vi "kalmanSeparatingObjects.vi"(1 "Detection Frame In":T1 {"robots_blue"."height" format="%+4.3f"; "robots_blue"."pixel_y" format="%+4.3f"; "robots_blue"."pixel_x" format="%+4.3f"; "robots_blue"."orientation" format="%+4.3f"; "robots_blue"."y" format="%+4.3f"; "robots_blue"."confidence" format="%4.3f"; "robots_blue"."x" format="%+4.3f"; "robots_yellow"."height" format="%+4.3f"; "robots_yellow"."pixel_y" format="%+4.3f"; "robots_yellow"."pixel_x" format="%+4.3f"; "robots_yellow"."orientation" format="%+4.3f"; "robots_yellow"."y" format="%+4.3f"; "robots_yellow"."confidence" format="%4.3f"; "robots_yellow"."x" format="%+4.3f"}, 3 "Time":enum16{"Azul", "Amarelo"}(ring) caption="Enum", 4 "Enable":bool) -> (15 "Detection Frame Out":T1 {"robots_blue"."height" format="%+4.3f"; "robots_blue"."pixel_y" format="%+4.3f"; "robots_blue"."pixel_x" format="%+4.3f"; "robots_blue"."orientation" format="%+4.3f"; "robots_blue"."y" format="%+4.3f"; "robots_blue"."confidence" format="%4.3f"; "robots_blue"."x" format="%+4.3f"; "robots_yellow"."height" format="%+4.3f"; "robots_yellow"."pixel_y" format="%+4.3f"; "robots_yellow"."pixel_x" format="%+4.3f"; "robots_yellow"."orientation" format="%+4.3f"; "robots_yellow"."y" format="%+4.3f"; "robots_yellow"."confidence" format="%4.3f"; "robots_yellow"."x" format="%+4.3f"})   [LabVIEW 2023, in "Vision.lvclass"]
uses:
  Vision.lvclass
  Old vision/Controls/SSL Detection Frame.ctl
  Old vision/Controls/SSL Detection Robot.ctl
  <vilib>/Analysis/Matrix/Datatypes/RealMatrix.ctl
  Old vision/Controls/SSL Detection Ball.ctl
  <vilib>/Analysis/Matrix/NI_Matrix.lvlib
panel:
  out "error out":errorcluster
  in  "error in (no error)":errorcluster
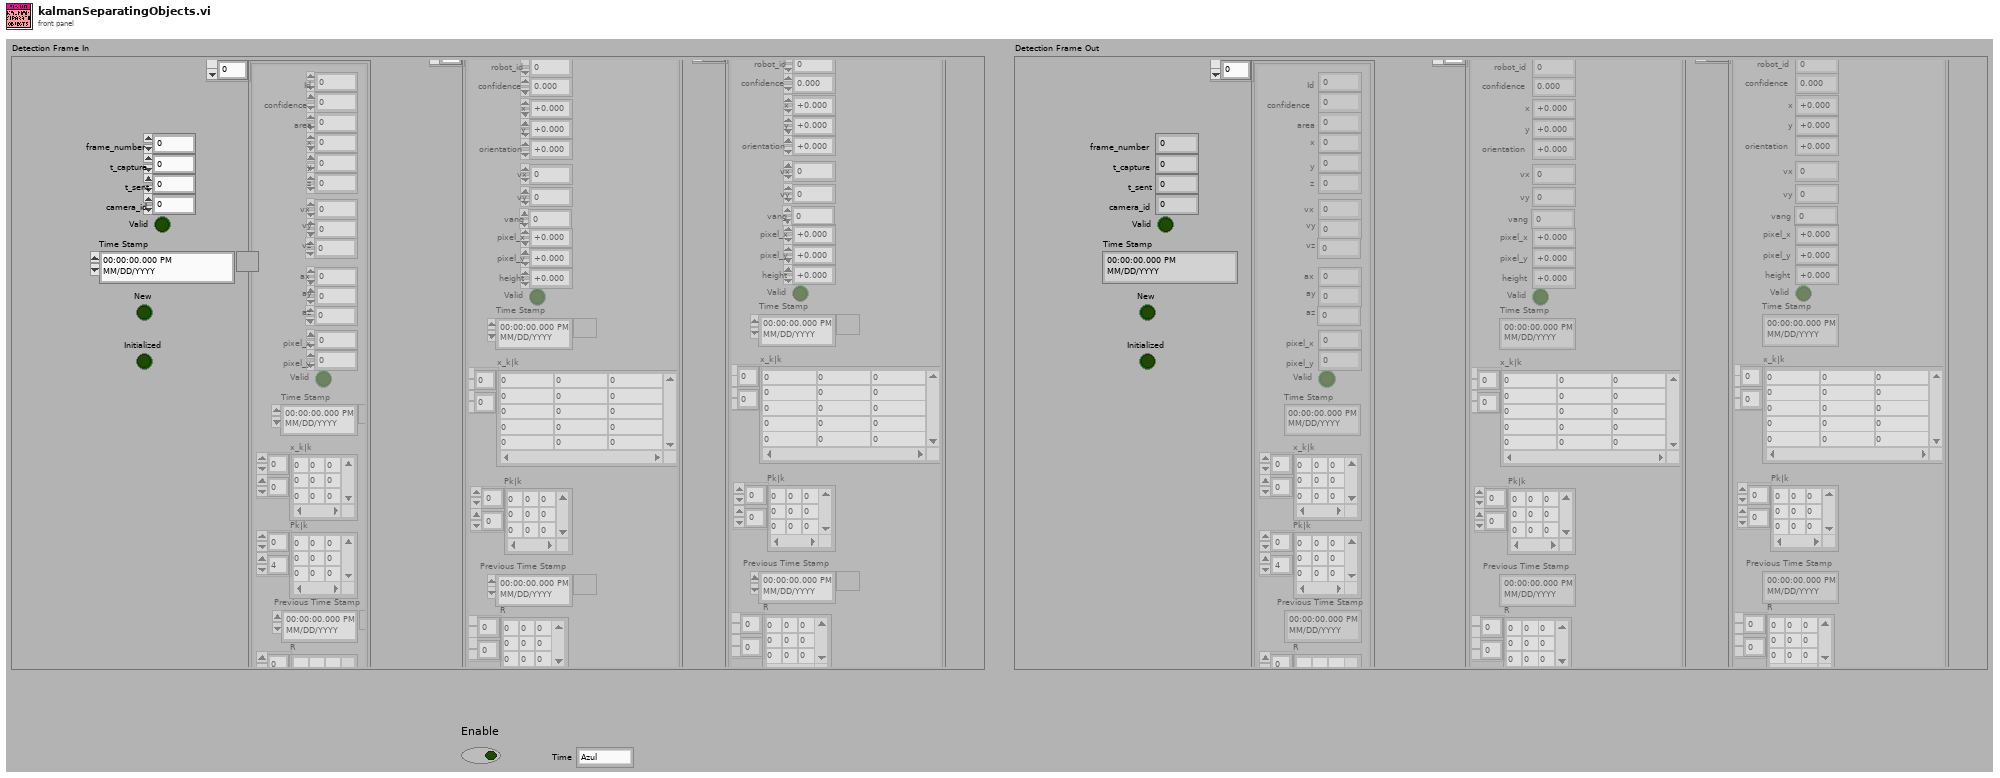
[diagram p1: front panel]
types:
  T1 = typedef "SSL Detection Frame.ctl" = cluster{"frame_number":u32, "t_capture":dbl, "t_sent":dbl, "camera_id":u32, "robots_yellow":T2[], "robots_blue":T2[], "balls":T4[], "Valid":bool, "Time Stamp":timestamp, "New":bool, "Initialized":bool}
  T2 = typedef "SSL Detection Robot.ctl" = cluster{"x":sgl, "robot_id":u32, "confidence":sgl, "y":sgl, "orientation":sgl, "pixel_x":sgl, "pixel_y":sgl, "height":sgl, "Valid":bool, "Time Stamp":timestamp, "x_k|k":T3, "Pk|k":T3, "Previous Time Stamp":timestamp, "R":T3, "vx":dbl, "vy":dbl, "vang":dbl}
  T3 = typedef "NI_Matrix.lvlib/RealMatrix.ctl" = dbl[][]
  T4 = typedef "SSL Detection Ball.ctl" = cluster{"x":sgl, "area":u32, "confidence":sgl, "y":sgl, "z":sgl, "pixel_x":sgl, "pixel_y":sgl, "Valid":bool, "Time Stamp":timestamp, "x_k|k":T3, "Pk|k":T3, "Id":u32, "Previous Time Stamp":timestamp, "R":T3, " vx":sgl, "vy":dbl, "vz":dbl, " ax":sgl, "ay":dbl, "az":dbl}
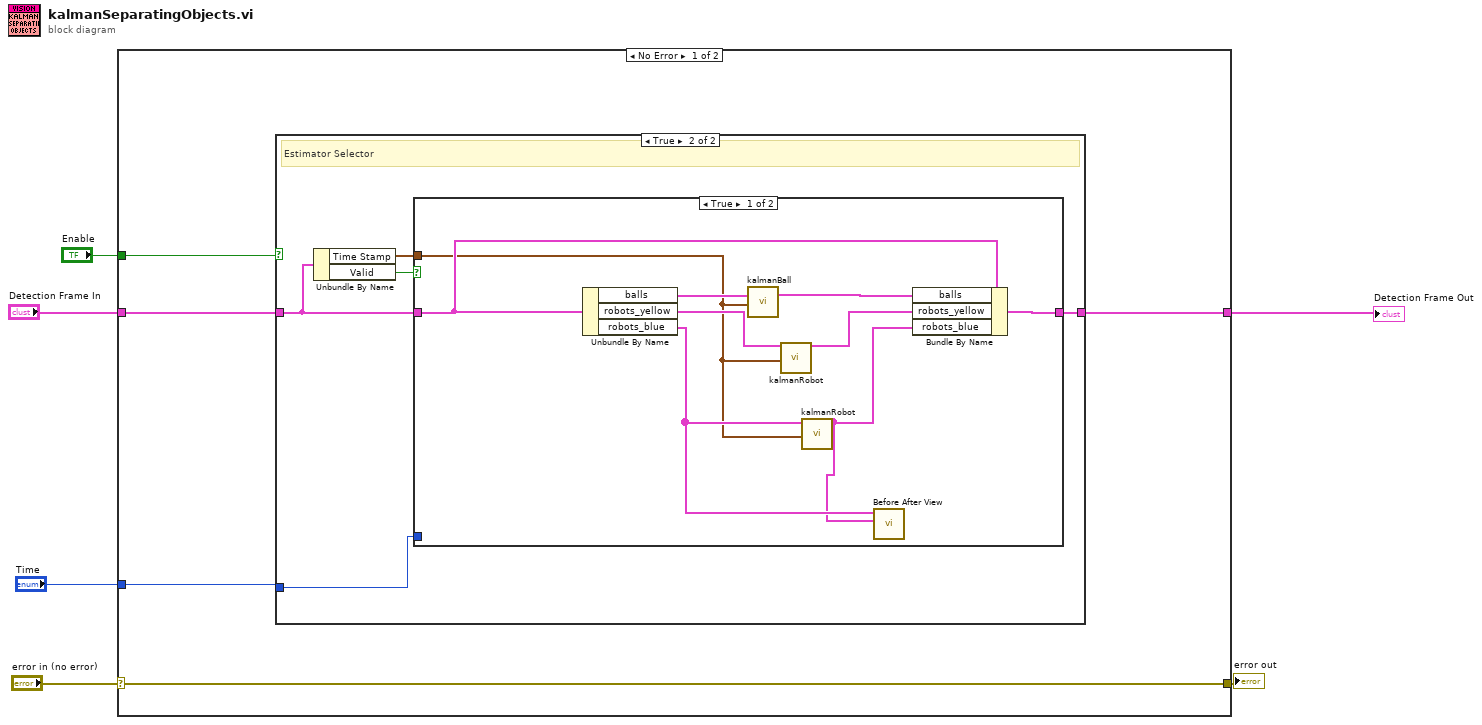
[diagram p0: block diagram]
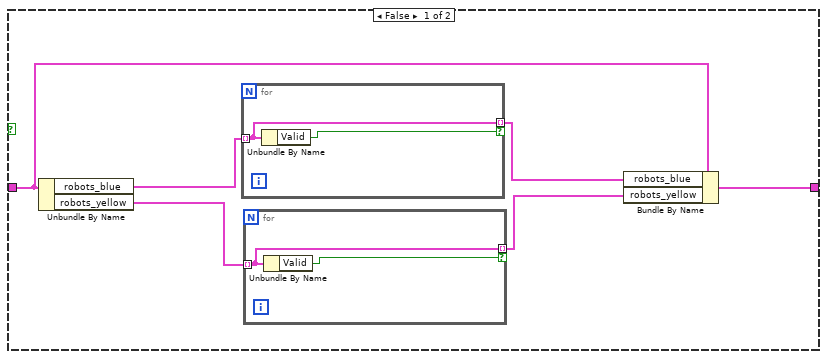
[diagram p2: hidden frame]
diagram:
  n1 = case shown="No Error" "error in (no error)" {
    selector: "error in (no error)" -> [w11 w37]
    tunnel: [w11 w37] -> w5
    tunnel: "Enable" -> [w10 _]
    tunnel: "Detection Frame In" -> [w9 _]
    tunnel: "Time" -> [w8 _]
    tunnel: [w7 _] -> w1
    frame No Error {
      n2 = case shown="True" w10 {
        tunnel: [w15 w26] -> w7
        tunnel: w9 -> [w16 w25]
        tunnel: w8 -> [_ w22]
        frame False {
          n3 = Unbundle By Name(w16) -> ("robots_blue"=w13:T2[], "robots_yellow"=w17:T2[])
          n4 = for {
            tunnel: w13 -> [w21] mode=indexing
            tunnel: [w21] -> w12 mode=indexing if=w20
            n5 = Unbundle By Name(w21) -> ("Valid"=w20:bool)
          }
          n6 = for {
            tunnel: w17 -> [w19] mode=indexing
            tunnel: [w19] -> w14 mode=indexing if=w18
            n7 = Unbundle By Name(w19) -> ("Valid"=w18:bool)
          }
          n8 = Bundle By Name(cluster=w16, "robots_blue"=w12, "robots_yellow"=w14) -> (w15:T1)
        }
        frame True {
          # "Estimator Selector"
          n9 = Unbundle By Name(w25) -> ("Time Stamp"=w23:timestamp, "Valid"=w24:bool)
          n10 = case shown="True" w24 {
            tunnel: w25 -> [w35 w36]
            tunnel: [w34 w36] -> w26
            tunnel: w23 -> [w27 _]
            tunnel: w22 -> [_ _]
            frame True {
              n11 = Unbundle By Name(w35) -> ("balls"=w33:T4[], "robots_yellow"=w31:T2[], "robots_blue"=w29:T2[])
              n12 = call "kalmanBall.vi"("Detection Ball \nArray"=w33, "Time Stamp 2"=w27) -> ("balls"=w32:T4[])  [unwired: 16 in, 1 out]
              n13 = call "kalmanRobot.vi"("robots_yellow in"=w31, "Time Stamp 2"=w27) -> ("robots_yellow out"=w30:T2[])  [unwired: 16 in, 1 out]
              n14 = call "kalmanRobot.vi"("robots_yellow in"=w29, "Time Stamp 2"=w27) -> ("robots_yellow out"=w28:T2[])  [unwired: 16 in, 1 out]
              n15 = call "Before After View.vi"("after"=w28, "before"=w29) -> ()  [unwired: 10 in]
              n16 = Bundle By Name(cluster=w35, "balls"=w32, "robots_yellow"=w30, "robots_blue"=w28) -> (w34:T1)
            }
            frame False {
            }
          }
        }
      }
    }
    frame Error {
    }
  }
  "error out" <- w5
  "Detection Frame Out" <- w1
